vi "Ion Sniffer.vi"() -> ()   [LabVIEW 2018]
uses:
  Type/_Source Type.ctl
  Type/_Log Command.ctl
  Type/_RT Command.ctl
  Type/_RT Instrument State.ctl
  Type/_SaveOption.ctl
  Type/_LC Command.ctl
  Configuration/_Global Configuration.vi
  <vilib>/Utility/config.llb/Read Key (Path).vi
  <vilib>/Utility/config.llb/Write Key (Path).vi
  <vilib>/Utility/config.llb/Read Key (String).vi
  <vilib>/Utility/config.llb/Write Key (String).vi
  Global.vi
  LCDriver/_Global LC Driver.vi
  <vilib>/Utility/config.llb/Read Key (I32).vi
  <vilib>/Utility/config.llb/Write Key (I32).vi
  <vilib>/Utility/miscctls.llb/LVRectTypeDef.ctl
  <vilib>/Utility/config.llb/NI_LVConfig.lvlib
panel:
  out "RT Events":string
  out "Exhaust OK":bool
  out "CurGas OK":bool
  out "Pump OK":bool
  out "Interlock OK":bool
  out "Vac. Pressure:":sgl format="%#.2e"
  out "HSID Temp:":sgl
  out "Source 2 Temp:":sgl
  out "Source 2 Type:":T1 items=["None", "ESI", "APCI", "APPI", "MicroSpray"]
  out "Source 1 Temp:":sgl
  out "Source 1 Type:":T1 items=["None", "ESI", "APCI", "APPI", "MicroSpray"]
  in  "Display":bool
  in  "Acquisition":bool
  in  "Tuning":bool
  in  "Diagnostics":bool
  in  "Configuration":bool
  # "Source Status"
  # "Other Status"
  # "Torr"
  # "Interlocks:"
  # "Pump Speed:"
  # "Curtain Gas:"
  # "Exhaust Gas:"
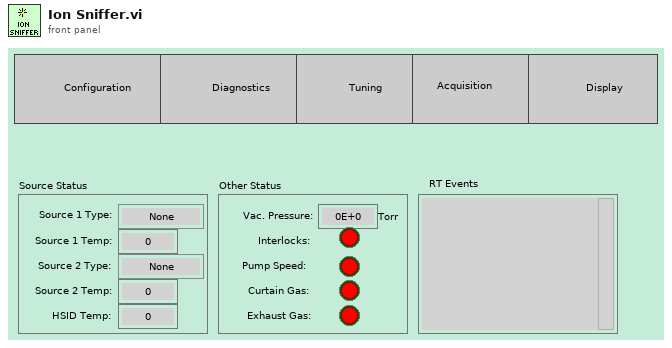
[diagram p1: front panel]
types:
  T1 = typedef "_Source Type.ctl" = i8
  T2 = typedef "_Log Command.ctl" = enum16{"No Command", "Open", "Read", "Write", "Close", "Check Size"}
  T3 = typedef "_RT Command.ctl" = enum16{"xml Start Run", "xml Start Actual Run", "xml Stop Run", "xml Runtime Update", "xml Get Status", "xml Get Table", "xml Set Table", "xml Get Configuration", "xml System Status", "xml Set LC Input Logic", "xml Get Data", "xml Get Info", "Start", "StartActualRun", "Stop", "Runtime Update", "Get Data", "Get Info", "Get Status", "Get Param", "Get Config", "Get Table", "Read ADC", "Set Oscillator", "Update Config", "Update Table", "Set All Pol", "Set Pol and DC", "Set Max Mass", "Toggle RP", "Toggle EL", "Set PIC", "Initialize Turbo", "Send Turbo Comm", "Close Turbo", "P1", "P2", "P3", "Send Serial", "Set LC Out", "Get LC In", "Read VAC", "Test Table", "Toggle Power", "Get Startup", "Set Startup", "Get ADC Table", "Set ADC Table", "Get Brief Status", "Get Detail Status", "Auxiliary Update", "Set CC Logics", "Set CC Input Logics", "Ignore Error", "invalid"}
  T4 = typedef "LVRectTypeDef.ctl" = cluster{"Left":i16, "Top":i16, "Right":i16, "Bottom":i16}
  T5 = typedef "_RT Instrument State.ctl" = enum16{"Initializing", "Mass Spectrometer is Off", "Starting Up", "Turning Power Off", "Going to Standby", "Roughing Pump Ready", "Turning Turbo Off", "Turbo Startup", "Turbopump Ready", "Checking Vacuum", "Going to Ready", "Ready", "Running", "Source Standby", "Lost Communication", "Shutting Down", "Fault", "24V Standby", "Go to 24V Standby", "Turbopump Ready-Waiting"}
  T6 = typedef "_SaveOption.ctl" = enum16{"Use Dialog", "Temporary File", "My Tables", "Full Path"}
  T7 = typedef "_LC Command.ctl" = enum16{"No Command", "Initialize", "Get Configuration", "Get Status", "Get LC Method Contents", "Oven OnOff", "Pump OnOFF", "Rinse Autosampler", "Run Sample", "Set EnvParameters", "Set Method", "Start Equilibration", "Stop Run", "Get LastError", "Clear Error", "Close"}
  T8 = typedef "NI_LVConfig.lvlib/Config Data RefNum.ctl" = refnum<k1>
  T9 = typedef "_LC Type.ctl" = enum16{"No LC", "Spark"}
  T10 = typedef "_RT Configuration 2.ctl" = cluster{"Name":string, "Ch#":u8, "Min":dbl, "Max":dbl, "Def+":dbl, "Def-":dbl, "Offset":dbl, "Slope":dbl, "Type":u8, "Description":string, "SettleT":dbl}
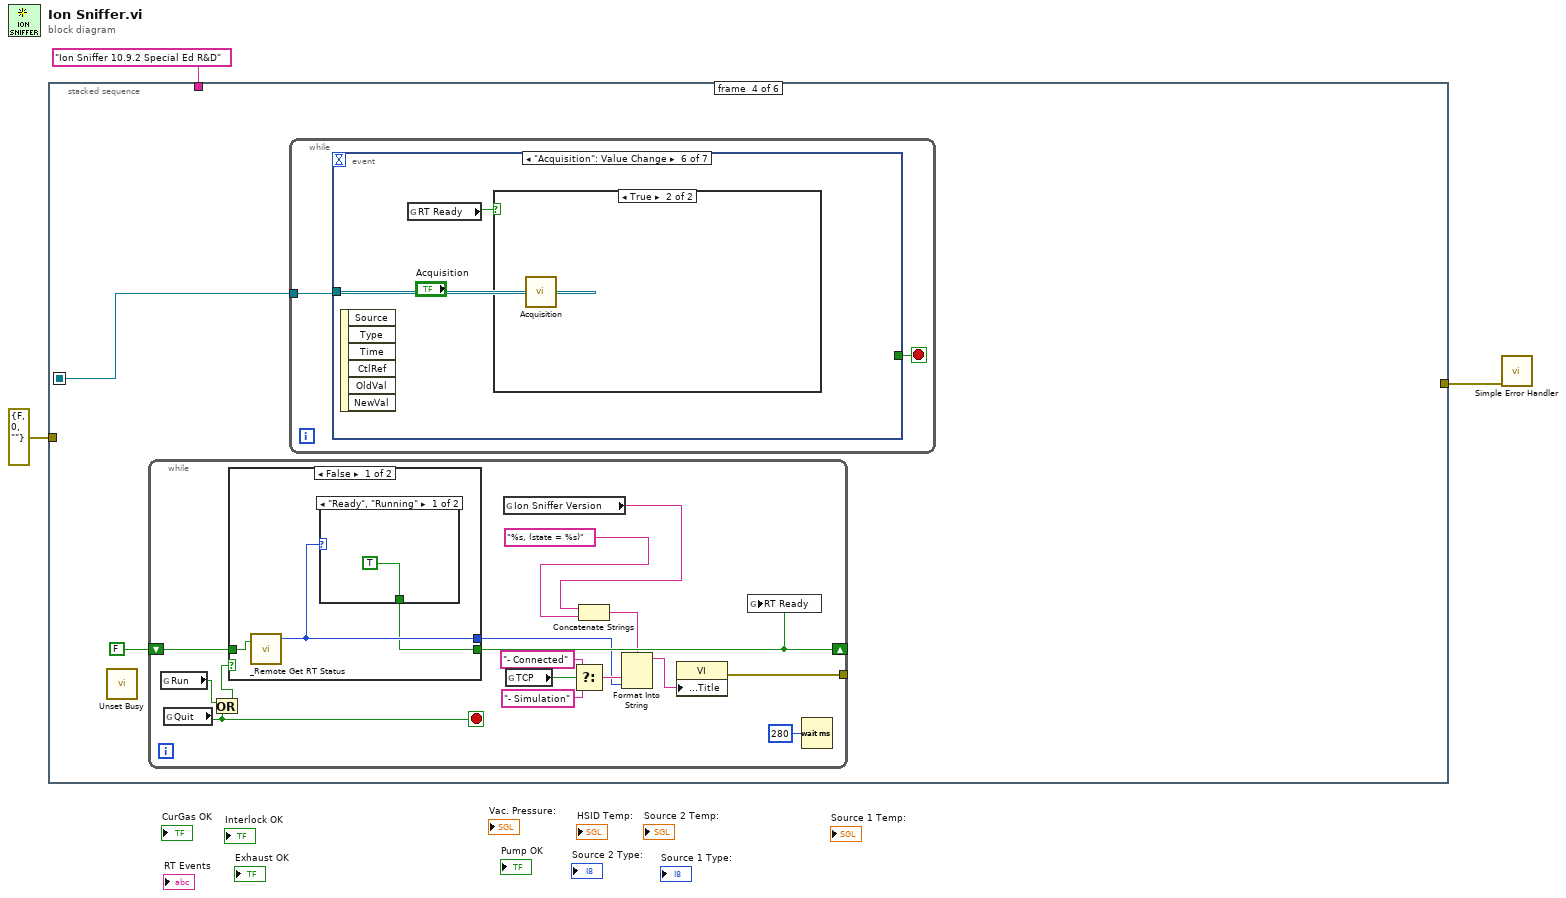
[diagram p0: block diagram]
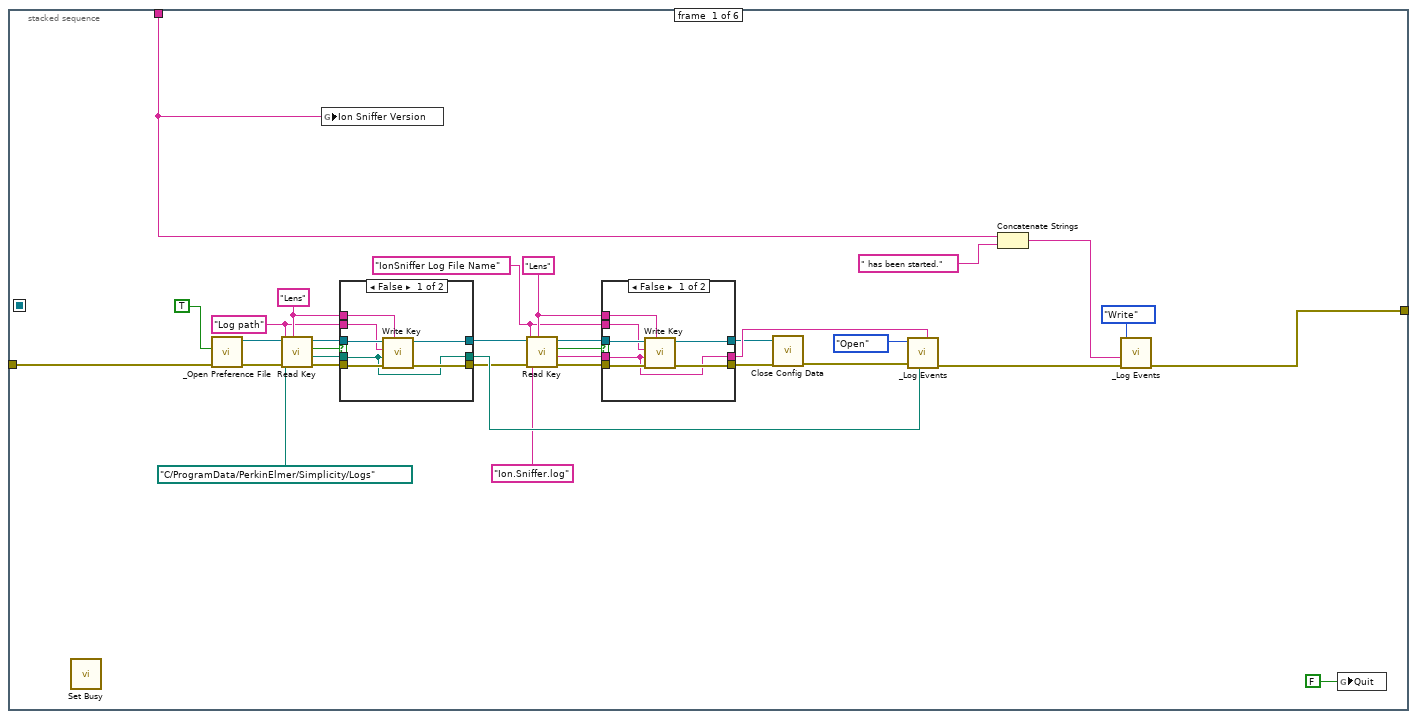
[diagram p2: hidden frame]
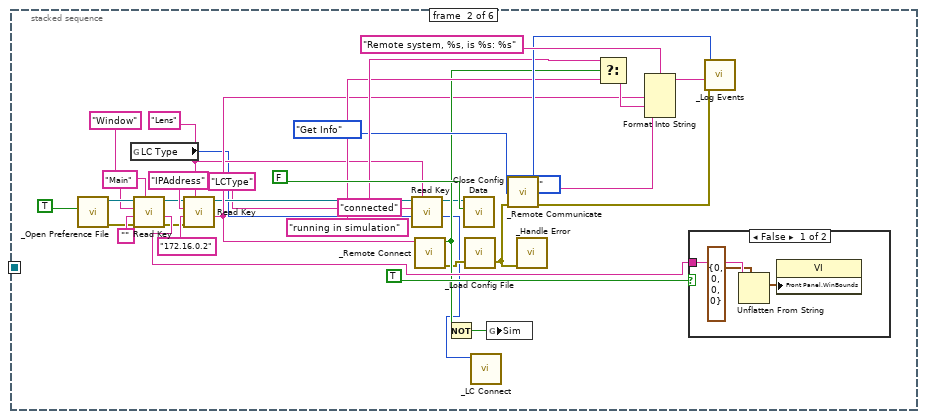
[diagram p5: hidden frame]
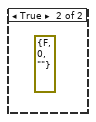
[diagram p6: hidden frame]
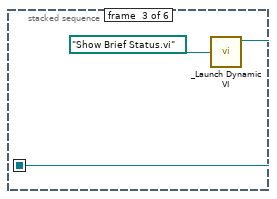
[diagram p7: hidden frame]
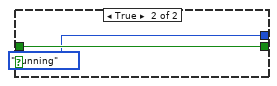
[diagram p9: hidden frame]
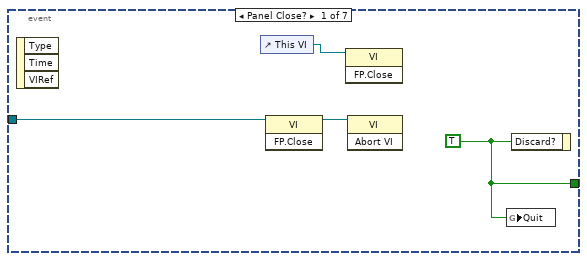
[diagram p10: hidden frame]
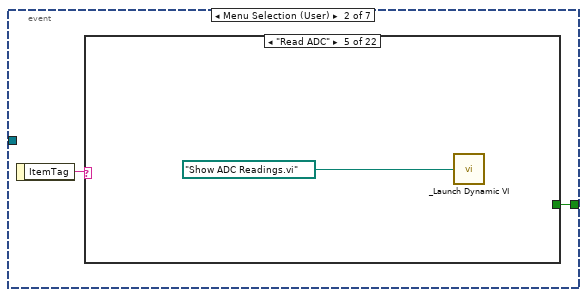
[diagram p11: hidden frame]
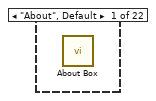
[diagram p12: hidden frame]
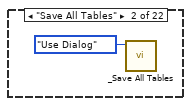
[diagram p13: hidden frame]
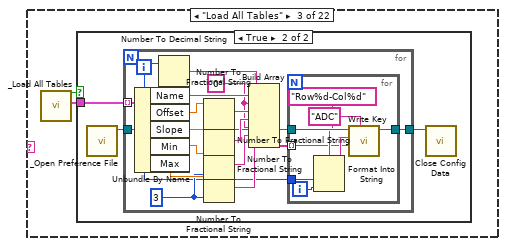
[diagram p14: hidden frame]
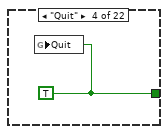
[diagram p16: hidden frame]
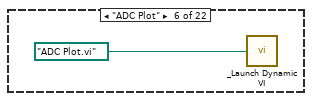
[diagram p17: hidden frame]
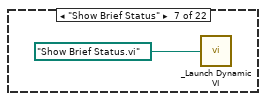
[diagram p18: hidden frame]
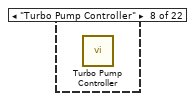
[diagram p19: hidden frame]
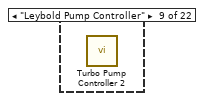
[diagram p20: hidden frame]
diagram:
  n1 = stacked-sequence {
    seq-local: [_ _ w93 _ _ _] -> [_ _ _ w95 _ _]
    tunnel: "Ion Sniffer 10.9.2 Special Ed R&D" ("string") -> [w8 _ _ _ _ _]
    tunnel: [w4 _ _ _ _ _] -> w2
    tunnel: errorcluster {"status"=FALSE, "code"=0, "source"=""} ("error constant") -> [w6 _ _ _ _ _]
    frame #0 {
      w13 = "IonSniffer Log File Name" ("key")
      w14 = "Lens" ("section")
      w19 = "Log path" ("key")
      w20 = "Lens" ("section")
      n2 = call <vilib>:"Set Busy.vi"() -> ()  [unwired: 4 in, 8 out]
      n3 = call "_Open Preference File.vi"("error In"=w6, "Initialize"=TRUE) -> ("error"=w28:errorcluster, "refnum"=w27:T8)  [unwired: 1 in, 3 out]
      n4 = call-poly <vilib>:"Read Key.vi"("section"=w20, "error in (no error)"=w28, "default value"=path "C:/ProgramData/PerkinElmer/Simplicity/Logs", "key"=w19, "refnum"=w27) -> ("error out"=w26:errorcluster, "value"=w24:path, "found?"=w25:bool, "refnum out"=w23:T8)  [unwired: 3 in]
      n5 = global write "Global.vi" "Ion Sniffer Version"(w8) -> ()
      n6 = case shown="False" w25 {
        tunnel: w26 -> [w53 w56]
        tunnel: w24 -> [w47 w54]
        tunnel: w23 -> [w51 w55]
        tunnel: [w52 w56] -> w22
        tunnel: [w50 w55] -> w21
        tunnel: [w47 w54] -> w34
        tunnel: w20 -> [w49 _]
        tunnel: w19 -> [w48 _]
        frame False {
          n7 = call-poly <vilib>:"Write Key.vi"("section"=w49, "error in (no error)"=w53, "value"=w47, "key"=w48, "refnum"=w51) -> ("error out"=w52:errorcluster, "refnum out"=w50:T8)  [unwired: 4 in, 1 out]
        }
        frame True {
        }
      }
      n8 = call-poly <vilib>:"Read Key.vi"("section"=w14, "error in (no error)"=w22, "default value"="Ion.Sniffer.log", "key"=w13, "refnum"=w21) -> ("error out"=w15:errorcluster, "value"=w16:string, "found?"=w17:bool, "refnum out"=w18:T8)  [unwired: 3 in]
      n9 = case shown="False" w17 {
        tunnel: w15 -> [w43 w46]
        tunnel: w16 -> [w37 w44]
        tunnel: w18 -> [w41 w45]
        tunnel: [w42 w46] -> w11
        tunnel: [w40 w45] -> w12
        tunnel: [w37 w44] -> w35
        tunnel: w14 -> [w39 _]
        tunnel: w13 -> [w38 _]
        frame False {
          n10 = call-poly <vilib>:"Write Key.vi"("section"=w39, "error in (no error)"=w43, "value"=w37, "key"=w38, "refnum"=w41) -> ("error out"=w42:errorcluster, "refnum out"=w40:T8)  [unwired: 4 in, 1 out]
        }
        frame True {
        }
      }
      n11 = call <vilib>:"Close Config Data.vi"("error in (no error)"=w11, "refnum"=w12) -> ("error out"=w5:errorcluster)  [unwired: 1 in, 8 out]
      n12 = call "_Log Events.vi"("File Name"=w35, "Log Path"=w34, "error in (no error)"=w5, "Log Command"=_Log_Command."Open" ("File Command")) -> ("error out"=w33:errorcluster)  [unwired: 4 in, 1 out]
      n13 = Concatenate Strings(w8, " has been started." ("string")) -> (w9:string)
      n14 = call "_Log Events.vi"("error in (no error)"=w33, "Event"=w9, "Log Command"=_Log_Command."Write" ("File Command")) -> ("error out"=w4:errorcluster)  [unwired: 5 in, 1 out]
      n15 = global write "_Global Configuration.vi" "Quit"(FALSE ("Quit")) -> ()
    }
    frame #1 {
      w64 = "Lens" ("section")
      n16 = call "_Open Preference File.vi"("Initialize"=TRUE) -> ("error"=w58:errorcluster, "refnum"=w84:T8)  [unwired: 2 in, 3 out]
      n17 = global read "_Global LC Driver.vi" "LC Type"() -> (w61:T9)
      n18 = call-poly <vilib>:"Read Key.vi"("section"="Window", "error in (no error)"=w58, "default value"="", "key"="Main" ("section"), "refnum"=w84) -> ("error out"=w57:errorcluster, "value"=w89:string, "refnum out"=w85:T8)  [unwired: 1 in, 3 out]
      n19 = call-poly <vilib>:"Read Key.vi"("section"=w64, "error in (no error)"=w57, "default value"="172.16.0.2", "key"="IPAddress" ("section"), "refnum"=w85) -> ("value"=w66:string, "refnum out"=w65:T8)  [unwired: 1 in, 4 out]
      n20 = call-poly <vilib>:"Read Key.vi"("section"=w64, "default value"=w61, "key"="LCType" ("section"), "refnum"=w65) -> ("value"=w60:i32, "refnum out"=w62:T8)  [unwired: 1 in, 5 out]
      n21 = call "_Remote Connect.vi"("IP Address"=w66) -> ("error out"=w69:errorcluster, "TCP"=w70:bool)  [unwired: 1 in, 4 out]
      n22 = Not(x=w70) -> (.not. x?=w71:bool)
      n23 = call <vilib>:"Close Config Data.vi"("write file if changed (T)"=FALSE ("write configuration file? (T)"), "refnum"=w62) -> ()  [unwired: 1 in, 9 out]
      n24 = call "_Load Config File.vi"("error in (no error)"=w69) -> ("error out"=w67:errorcluster)  [unwired: 1 in, 1 out]
      n25 = call "_LC Connect.vi"("LC Type"=w60) -> ()  [unwired: 7 out]
      n26 = global write "_Global Configuration.vi" "Sim"(w71) -> ()
      n27 = call "_Remote Communicate.vi"("error in (no error)"=w67, "Command"=_RT_Command."Get Info") -> ("error out"=w68:errorcluster, "Info"=w72:string)  [unwired: 4 in, 2 out]
      n28 = call "_Handle Error.vi"("error in (no error)"=w67) -> ()  [unwired: 2 in, 5 out]
      n29 = Select(t="connected", s=w70, f="running in simulation") -> (s? t:f=w78:string)
      n30 = Format Into String(format string="Remote system, %s, is %s: %s", w66, w78, w72) -> (resulting string=w77:string)  [unwired: 2 in, 1 out]
      n31 = case shown="False" TRUE {
        tunnel: w89 -> [w92 _]
        frame False {
          n32 = Unflatten From String(type=T4 {"Left"=0, "Top"=0, "Right"=0, "Bottom"=0} ("Front Panel Window:Window Bounds"), binary string=w92) -> (value=w90:T4)  [unwired: 1 in, 4 out]
          n33 = property class="VI"("Front Panel.WinBounds"=w90) -> ()  [unwired: 2 in, 2 out]
        }
        frame True {
          (unwired) errorcluster {"status"=FALSE, "code"=0, "source"=""} ("error constant")
        }
      }
      n34 = call "_Log Events.vi"("error in (no error)"=w68, "Event"=w77, "Log Command"=_Log_Command."Write" ("File Command")) -> ()  [unwired: 5 in, 2 out]
    }
    frame #2 {
      n35 = call "_Launch Dynamic VI.vi"("VI Name"=path "Show Brief Status.vi" ("name or relative path")) -> ("VI Refnum"=w93:refnum<vi>)  [unwired: 3 in]
    }
    frame #3 {
      n36 = call <vilib>:"Unset Busy.vi"() -> ()  [unwired: 2 in, 10 out]
      n37 = while {
        shift-right: [w105] -> _
        shift-left: FALSE -> [w112]
        tunnel: [w97] -> _
        stop <- w103 stop-if-true
        n38 = global read "_Global Configuration.vi" "Run"() -> (w102:bool)
        n39 = global read "_Global Configuration.vi" "Quit"() -> (w103:bool)
        n40 = Or(x=w102, y=w103) -> (x .or. y?=w101:bool)
        n41 = case shown="False" w101 {
          tunnel: w112 -> [w115 w118]
          tunnel: [w114 _RT_Instrument_State."Running" ("InstrState")] -> w104
          tunnel: [w113 w118] -> w105
          frame False {
            n42 = call "_Remote Get RT Status.vi"("RT Ready"=w115) -> ("InstrState"=w114:T5)  [unwired: 1 in, 2 out]
            n43 = case shown="\"Ready\", \"Running\"" w114 {
              tunnel: [TRUE _] -> w113
              frame "Ready", "Running" {
              }
              frame Default {
              }
            }
          }
          frame True {
          }
        }
        n44 = global read "Global.vi" "Ion Sniffer Version"() -> (w98:string)
        n45 = global read "_Global Configuration.vi" "TCP"() -> (w109:bool)
        n46 = Select(t="- Connected", s=w109, f="- Simulation") -> (s? t:f=w106:string)
        n47 = Concatenate Strings(w98, "%s, (state = %s)" ("string")) -> (w100:string)
        n48 = Format Into String(format string=w100, w106, w104) -> (resulting string=w110:string)  [unwired: 2 in, 1 out]
        n49 = property class="VI"("Front Panel Window:Title"=w110) -> (error out=w97:errorcluster)  [unwired: 2 in, 1 out]
        n50 = global write "_Global Configuration.vi" "RT Ready"(w105) -> ()
        n51 = Wait (ms)(milliseconds to wait=u32 280) -> ()  [unwired: 1 out]
      }
      n52 = while {
        tunnel: w95 -> [w119]
        stop <- w120 stop-if-true
        n53 = event shown="[5] \"Acquisition\": Value Change" {
          selector: _ -> [_ _ _ _ _ _ _]
          dyn-events: _ -> [_ _ _ _ _ _ _]
          timeout: _ -> [_ _ _ _ _ _ _]
          tunnel: [w124 w125 _ _ _ _ _] -> w120
          tunnel: w119 -> [w122 _ _ _ _ _ _]
          event Panel Close? {
            w124 = TRUE
            n54 = event-data() -> ()  [unwired: 4 out]
            n55 = control-ref of="This VI"() -> (w123:refnum<vi>)
            n56 = invoke class="VI" method="FP.Close"(reference=w122) -> (reference out=w121:refnum<vi>)  [unwired: 2 in, 2 out]
            n57 = invoke class="VI" method="FP.Close"(reference=w123) -> ()  [unwired: 2 in, 3 out]
            n58 = invoke class="VI" method="Abort VI"(reference=w121) -> ()  [unwired: 2 in, 3 out]
            n59 = global write "_Global Configuration.vi" "Quit"(w124) -> ()
            n60 = event-data("Discard?"=w124) -> ()  [unwired: 1 in, 1 out]
          }
          event Menu Selection (User) {
            n61 = event-data() -> ("ItemTag"=w126:string)  [unwired: 1 out]
            n62 = case shown="\"Read ADC\"" w126 {
              tunnel: [_ _ _ w158 _ _ _ _ _ _ _ _ _ _ _ _ _ _ _ _ _ _] -> w125
              frame "About", Default {
                n63 = call "About Box.vi"() -> ()  [unwired: 1 out]
              }
              frame "Save All Tables" {
                n64 = call "_Save All Tables.vi"("SaveOption (Temporary File)"=_SaveOption."Use Dialog") -> ()  [unwired: 2 in, 5 out]
              }
              frame "Load All Tables" {
                n65 = call "_Load All Tables.vi"() -> ("ADC Table"=w128:T10[], "Loaded ADC"=w129:bool)  [unwired: 1 in, 5 out]
                n66 = case shown="True" w129 {
                  tunnel: w128 -> [_ w132]
                  frame False {
                  }
                  frame True {
                    n67 = call "_Open Preference File.vi"() -> ("refnum"=w131:T8)  [unwired: 3 in, 4 out]
                    n68 = for {
                      tunnel: w132 -> [w149] mode=indexing
                      tunnel: w131 -> [w136]
                      tunnel: [w134] -> w130
                      i -> [w135]
                      w139 = "0"
                      w144 = i16 3 ("precision (6)")
                      n69 = Unbundle By Name(w149) -> ("Name"=w142:string, "Offset"=w148:dbl, "Slope"=w147:dbl, "Min"=w146:dbl, "Max"=w145:dbl)
                      n70 = Number To Decimal String(number=w135) -> (decimal integer string=w143:string)  [unwired: 1 out]
                      n71 = Number To Fractional String(number=w148) -> (F-format string=w141:string)  [unwired: 3 out]
                      n72 = Number To Fractional String(number=w147) -> (F-format string=w140:string)  [unwired: 3 out]
                      n73 = Number To Fractional String(number=w146, precision (6)=w144) -> (F-format string=w138:string)  [unwired: 2 out]
                      n74 = Number To Fractional String(number=w145, precision (6)=w144) -> (F-format string=w137:string)  [unwired: 2 out]
                      n75 = Build Array(w143, w142, w139, w141, w140, w139, w138, w137) -> (w133:string[])
                      n76 = for {
                        tunnel: w136 -> [w157]
                        tunnel: [w156] -> w134
                        tunnel: w135 -> [w154]
                        tunnel: w133 -> [w150] mode=indexing
                        i -> [w155]
                        n77 = Format Into String(format string="Row%d-Col%d" ("section"), w154, w155) -> (resulting string=w152:string)  [unwired: 2 in, 1 out]
                        n78 = call-poly <vilib>:"Write Key.vi"("section"="ADC", "value"=w150, "key"=w152, "refnum"=w157) -> ("refnum out"=w156:T8)  [unwired: 2 in, 5 out]
                      }
                    }
                    n79 = call <vilib>:"Close Config Data.vi"("refnum"=w130) -> ()  [unwired: 2 in, 9 out]
                  }
                }
              }
              frame "Quit" {
                w158 = TRUE
                n80 = global write "_Global Configuration.vi" "Quit"(w158) -> ()
              }
              frame "Read ADC" {
                n81 = call "_Launch Dynamic VI.vi"("VI Name"=path "Show ADC Readings.vi" ("name or relative path")) -> ()  [unwired: 3 in, 1 out]
              }
              frame "ADC Plot" {
                n82 = call "_Launch Dynamic VI.vi"("VI Name"=path "ADC Plot.vi" ("name or relative path")) -> ()  [unwired: 3 in, 1 out]
              }
              frame "Show Brief Status" {
                n83 = call "_Launch Dynamic VI.vi"("VI Name"=path "Show Brief Status.vi" ("name or relative path")) -> ()  [unwired: 3 in, 1 out]
              }
              frame "Turbo Pump Controller" {
                n84 = call "Turbo Pump Controller.vi"() -> ()  [unwired: 8 out]
              }
              frame "Leybold Pump Controller" {
                n85 = call "Turbo Pump Controller 2.vi"() -> ()  [unwired: 8 in]
              }
              frame "Syringe Pump Controller" {
                n86 = call "Syringe Pump Controller.vi"() -> ()  [unwired: 8 out]
              }
              frame "LCD Controller" {
                n87 = call "LCD Controller.vi"() -> ()  [unwired: 8 out]
              }
              frame "Start-Up Options" {
                n88 = call "Start Up Options.vi"() -> ()  [unwired: 1 in, 7 out]
              }
              frame "Source Controller" {
                n89 = call "Source Controller.vi"() -> ()  [unwired: 8 out]
              }
              frame "Serial Test Controller" {
                n90 = call "Serial Test Controller.vi"() -> ()  [unwired: 8 out]
              }
              frame "Read FPGA Map" {
                n91 = call "Show FPGA Map.vi"() -> ()  [unwired: 12 out]
              }
              frame "Test Table" {
                n92 = call "Table Test.vi"() -> ()  [unwired: 1 out]
              }
              frame "Re-Connect" {
                n93 = stacked-sequence {
                  tunnel: [_ w165 _] -> w162
                  frame #0 {
                    n94 = call <vilib>:"Set Busy.vi"() -> ()  [unwired: 4 in, 8 out]
                  }
                  frame #1 {
                    n95 = call "_Open Preference File.vi"() -> ("error"=w163:errorcluster, "refnum"=w164:T8)  [unwired: 3 in, 3 out]
                    n96 = call-poly <vilib>:"Read Key.vi"("section"="Lens", "error in (no error)"=w163, "default value"="172.16.0.2", "key"="IPAddress" ("section"), "refnum"=w164) -> ("error out"=w169:errorcluster, "value"=w167:string, "refnum out"=w170:T8)  [unwired: 1 in, 3 out]
                    n97 = call <vilib>:"Close Config Data.vi"("error in (no error)"=w169, "write file if changed (T)"=FALSE ("write configuration file? (T)"), "refnum"=w170) -> ()  [unwired: 9 out]
                    n98 = call "_Remote Connect.vi"("IP Address"=w167) -> ("error out"=w166:errorcluster)  [unwired: 1 in, 5 out]
                    n99 = call "_Load Config File.vi"("error in (no error)"=w166) -> ("error out"=w165:errorcluster)  [unwired: 1 in, 1 out]
                  }
                  frame #2 {
                    n100 = call <vilib>:"Unset Busy.vi"() -> ()  [unwired: 2 in, 10 out]
                  }
                }
                n101 = call "_Handle Error.vi"("error in (no error)"=w162) -> ()  [unwired: 2 in, 5 out]
              }
              frame "mzData Converter" {
                n102 = call "_mzData Converter.vi"() -> ()  [unwired: 2 out]
              }
              frame "txtData Converter" {
                n103 = call "_txtData Converter.vi"() -> ()  [unwired: 2 out]
              }
              frame "Start System" {
                n104 = call "_Remote Communicate.vi"("DC Param"=u16 0, "Command"=_RT_Command."Toggle Power") -> ("error out"=w174:errorcluster)  [unwired: 4 in, 3 out]
                n105 = call <vilib>:"Simple Error Handler.vi"("error in (no error)"=w174) -> ()  [unwired: 1 in, 8 out]
              }
              frame "Goto Roughing Pump On Standby" {
                n106 = call "_Remote Communicate.vi"("DC Param"=u16 1, "Command"=_RT_Command."Toggle Power") -> ("error out"=w177:errorcluster)  [unwired: 4 in, 3 out]
                n107 = call <vilib>:"Simple Error Handler.vi"("error in (no error)"=w177) -> ()  [unwired: 1 in, 8 out]
              }
              frame "Shut Down System" {
                n108 = call "_Remote Communicate.vi"("DC Param"=u16 2, "Command"=_RT_Command."Toggle Power") -> ("error out"=w180:errorcluster)  [unwired: 4 in, 3 out]
                n109 = call <vilib>:"Simple Error Handler.vi"("error in (no error)"=w180) -> ()  [unwired: 1 in, 8 out]
              }
            }
          }
          event "Configuration": Value Change {
            n110 = event-data() -> ()  [unwired: 7 out]
            n111 = call "Edit Configuration.vi"() -> ()  [unwired: 8 out]
          }
          event "Diagnostics": Value Change {
            n112 = event-data() -> ()  [unwired: 7 out]
            n113 = call "Diagnostic.vi"() -> ()  [unwired: 8 out]
          }
          event "Tuning": Value Change {
            n114 = event-data() -> ()  [unwired: 7 out]
            n115 = global read "_Global Configuration.vi" "RT Ready"() -> (w183:bool)
            n116 = case shown="True" w183 {
              frame False {
                n117 = One Button Dialog(message="System is not ready.") -> ()  [unwired: 2 out]
              }
              frame True {
                n118 = call "Tuning.vi"() -> ()  [unwired: 8 out]
              }
            }
          }
          event "Acquisition": Value Change {
            n119 = event-data() -> ()  [unwired: 7 out]
            n120 = global read "_Global Configuration.vi" "RT Ready"() -> (w185:bool)
            n121 = case shown="True" w185 {
              frame False {
                n122 = One Button Dialog(message="System is not ready.") -> ()  [unwired: 2 out]
              }
              frame True {
                n123 = call "Acquisition.vi"() -> ()  [unwired: 8 out]
              }
            }
          }
          event "Display": Value Change {
            n124 = event-data() -> ()  [unwired: 7 out]
            n125 = call "Data Viewer.vi"() -> ()  [unwired: 1 out]
          }
        }
      }
    }
    frame #4 {
      n126 = call "_LC Send Command.vi"("Command"=_LC_Command."Close") -> ("error out"=w187:errorcluster)  [unwired: 9 in, 1 out]
      n127 = call "_Remote Communicate.vi"("error in (no error)"=w187, "DC Param"=u16 1, "Command"=_RT_Command."Ignore Error") -> ()  [unwired: 3 in, 4 out]
    }
    frame #5 {
      n128 = property class="VI"() -> (error out=w193:errorcluster, "Front Panel.WinBounds"=w203:T4)  [unwired: 2 in, 1 out]
      n129 = Flatten To String(anything=w203, error in (no error)=w193) -> (data string=w202:string, error out=w192:errorcluster)  [unwired: 3 out]
      n130 = call "_Open Preference File.vi"("error In"=w192) -> ("error"=w206:errorcluster, "refnum"=w207:T8)  [unwired: 2 in, 3 out]
      n131 = global read "_Global LC Driver.vi" "LC Type"() -> (w196:T9)
      n132 = call-poly <vilib>:"Write Key.vi"("section"="Window", "error in (no error)"=w206, "value"=w202, "key"="Main" ("section"), "refnum"=w207) -> ("error out"=w200:errorcluster, "refnum out"=w199:T8)  [unwired: 1 in, 4 out]
      n133 = call-poly <vilib>:"Write Key.vi"("section"="Lens", "error in (no error)"=w200, "value"=w196, "key"="LCType" ("section"), "refnum"=w199) -> ("error out"=w194:errorcluster, "refnum out"=w195:T8)  [unwired: 5 out]
      n134 = call <vilib>:"Close Config Data.vi"("error in (no error)"=w194, "refnum"=w195) -> ("error out"=w191:errorcluster)  [unwired: 1 in, 8 out]
      n135 = call "_Log Events.vi"("error in (no error)"=w191, "Log Command"=_Log_Command."Close" ("File Command")) -> ()  [unwired: 6 in, 2 out]
    }
  }
  n136 = call <vilib>:"Simple Error Handler.vi"("error in (no error)"=w2) -> ()  [unwired: 4 in, 5 out]
